vi "Core_QDSM.vi"() -> ()   [LabVIEW 2018]
panel:
  out "Numeric Display":cdb
  in  "Standard":bool
  in  "Complex":bool
  in  "Stop":bool
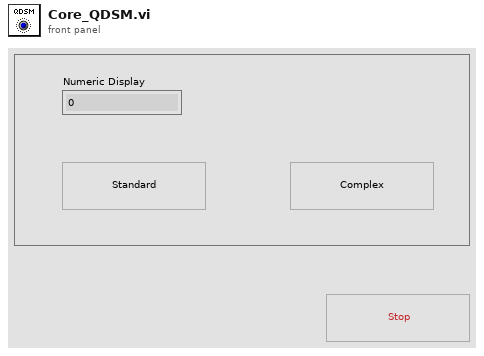
[diagram p1: front panel]
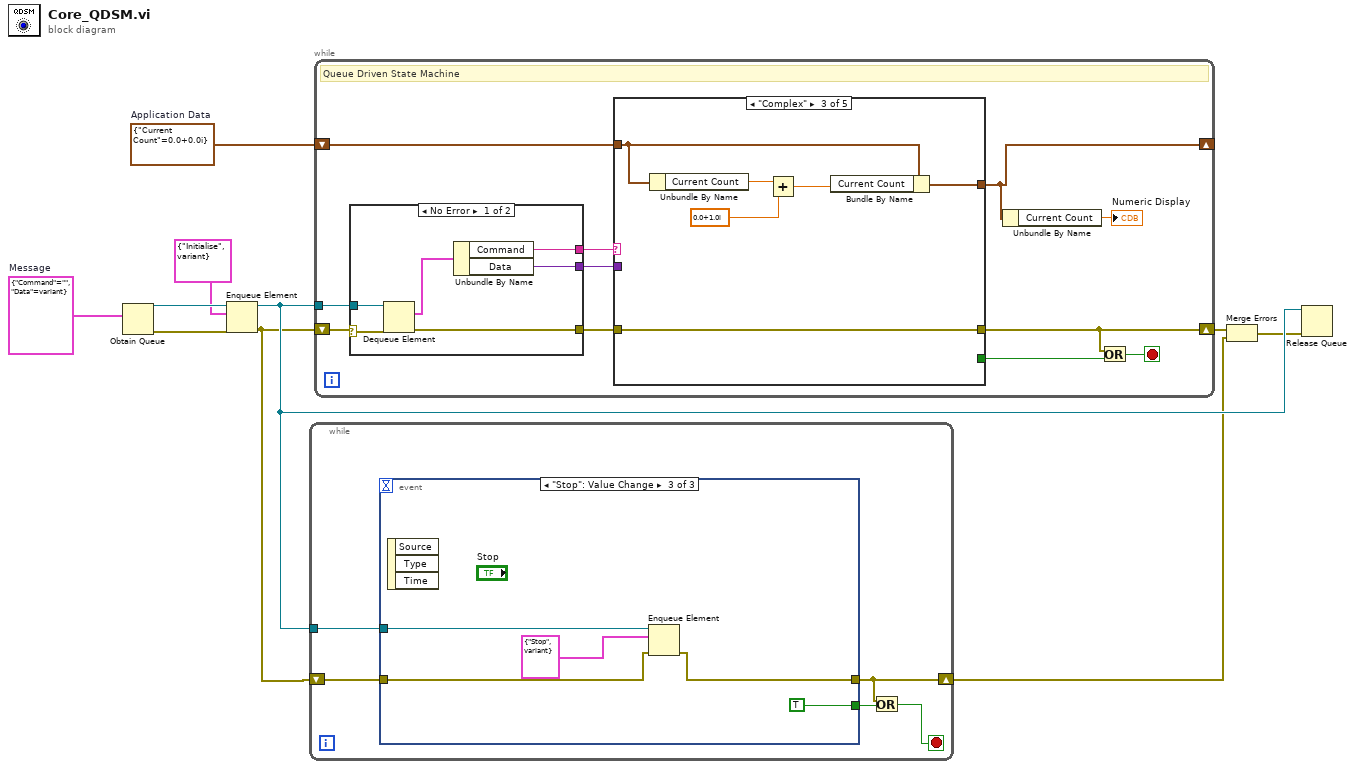
[diagram p0: block diagram]
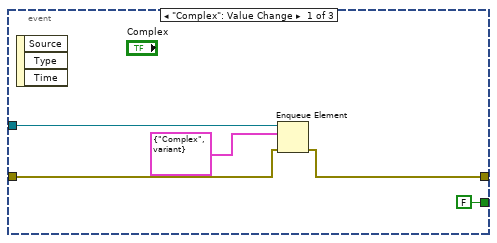
[diagram p2: hidden frame]
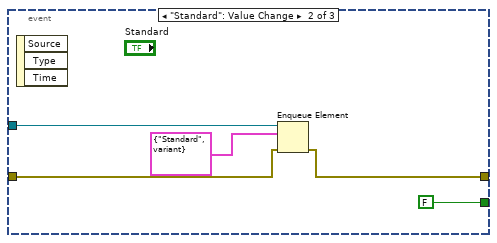
[diagram p3: hidden frame]
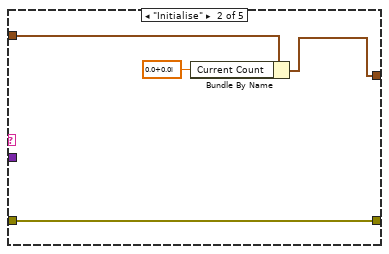
[diagram p5: hidden frame]
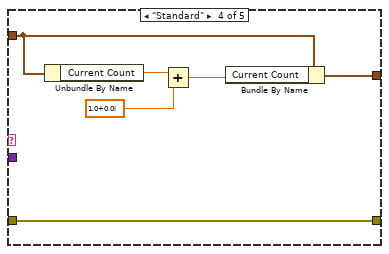
[diagram p6: hidden frame]
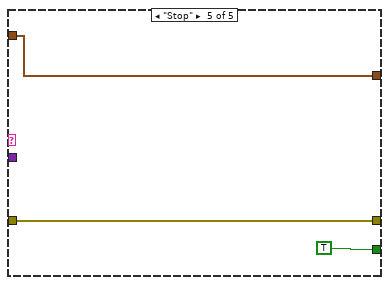
[diagram p7: hidden frame]
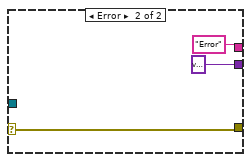
[diagram p8: hidden frame]
diagram:
  w1 = cluster{"Current Count":cdb} {"Current Count"=0.0+0.0i}  # Application Data
  w9 = cluster{"Command":string, "Data":variant} {"Command"="", "Data"=variant}  # Message
  n1 = Obtain Queue(element data type=w9) -> (queue out=w10:refnum<queue>, error out=w8:errorcluster)  [unwired: 4 in, 1 out]
  n2 = Enqueue Element(queue=w10, element=cluster{"Command":string, "Data":variant} {"Command"="Initialise", "Data"=variant}, error in (no error)=w8) -> (queue out=w6:refnum<queue>, error out=w5:errorcluster)  [unwired: 1 in, 1 out]
  n3 = while {
    tunnel: w6 -> [w15]
    shift-right: [w13] -> w3
    shift-left: w5 -> [w14]
    stop <- w11 stop-if-true
    n4 = event shown="[2] \"Stop\": Value Change" {
      selector: _ -> [_ _ _]
      dyn-events: _ -> [_ _ _]
      timeout: _ -> [_ _ _]
      tunnel: w15 -> [w20 w25 w30]
      tunnel: w14 -> [w18 w23 w28]
      tunnel: [w17 w22 w27] -> w13
      tunnel: [FALSE FALSE TRUE] -> w12
      event "Complex": Value Change {
        n5 = event-data() -> ()  [unwired: 1 in, 3 out]
        n6 = Enqueue Element(queue=w20, element=cluster{"Command":string, "Data":variant} {"Command"="Complex", "Data"=variant}, error in (no error)=w18) -> (error out=w17:errorcluster)  [unwired: 1 in, 2 out]
      }
      event "Standard": Value Change {
        n7 = event-data() -> ()  [unwired: 1 in, 3 out]
        n8 = Enqueue Element(queue=w25, element=cluster{"Command":string, "Data":variant} {"Command"="Standard", "Data"=variant}, error in (no error)=w23) -> (error out=w22:errorcluster)  [unwired: 1 in, 2 out]
      }
      event "Stop": Value Change {
        n9 = event-data() -> ()  [unwired: 1 in, 3 out]
        n10 = Enqueue Element(queue=w30, element=cluster{"Command":string, "Data":variant} {"Command"="Stop", "Data"=variant}, error in (no error)=w28) -> (error out=w27:errorcluster)  [unwired: 1 in, 2 out]
      }
    }
    n11 = Or(x=w13, y=w12) -> (x .or. y?=w11:bool)
  }
  n12 = while {
    tunnel: w6 -> [w40]
    shift-right: [w33] -> w4
    shift-left: w5 -> [w41]
    shift-right: [w35] -> _
    shift-left: w1 -> [w36]
    stop <- w31 stop-if-true
    # "Queue Driven State Machine"
    n13 = case shown="No Error" w41 {
      selector: w41 -> [w67 w71]
      tunnel: w40 -> [w68 _]
      tunnel: [w65 w71] -> w37
      tunnel: [w64 "Error" ("Command")] -> w39
      tunnel: [w63 variant ("Data")] -> w38
      frame No Error {
        n14 = Dequeue Element(queue=w68, error in (no error)=w67) -> (element=w66:cluster{"Command":string, "Data":variant}, error out=w65:errorcluster)  [unwired: 1 in, 2 out]
        n15 = Unbundle By Name(w66) -> ("Command"=w64:string, "Data"=w63:variant)
      }
      frame Error {
      }
    }
    n16 = case shown="\"Complex\"" w39 {
      tunnel: w38 -> [_ _ _ _ _]
      tunnel: w37 -> [w43 w47 w48 w54 w61]
      tunnel: [w43 w47 w48 w54 w61] -> w33
      tunnel: w36 -> [w42 w46 w51 w57 w62]
      tunnel: [w42 w44 w49 w55 w62] -> w35
      tunnel: [_ _ _ _ TRUE] -> w32
      frame "Error", Default {
      }
      frame "Initialise" {
        n17 = Bundle By Name(cluster=w46, "Current Count"=cdb 0.0+0.0i) -> (w44:cluster{"Current Count":cdb})
      }
      frame "Complex" {
        n18 = Unbundle By Name(w51) -> ("Current Count"=w53:cdb)
        n19 = Add(x=w53, y=cdb 0.0+1.0i) -> (x+y=w50:cdb)
        n20 = Bundle By Name(cluster=w51, "Current Count"=w50) -> (w49:cluster{"Current Count":cdb})
      }
      frame "Standard" {
        n21 = Unbundle By Name(w57) -> ("Current Count"=w59:cdb)
        n22 = Add(x=w59, y=cdb 1.0+0.0i) -> (x+y=w56:cdb)
        n23 = Bundle By Name(cluster=w57, "Current Count"=w56) -> (w55:cluster{"Current Count":cdb})
      }
      frame "Stop" {
      }
    }
    n24 = Unbundle By Name(w35) -> ("Current Count"=→"Numeric Display":cdb)
    n25 = Or(x=w33, y=w32) -> (x .or. y?=w31:bool)
  }
  n26 = Merge Errors(w4, w3) -> (w2:errorcluster)
  n27 = Release Queue(queue=w6, error in (no error)=w2) -> ()  [unwired: 1 in, 3 out]
